vi "I2C_IRQNotifyHost.vi"(8 "error out in":errorcluster, 10 "IRQ Number":u8) -> (0 "error out":errorcluster, 2 "i2c_State":T1)   [LabVIEW 2019]
doc: "Notifies the Host via IRQ that the I2C task has been completed, not that it was successful but that the task has completed executing.\n\n<b>Inputs:</b>\n---------------------\n<b>IRQ Number</b> the IRQ number used for notification.\n0 Write\n1 Read\n3 Write w/Read\n\n<b>Outputs:</b>\n---------------------\n<b>i2c_State</b> hard coded to 'Monitor'\n\nSee block diagram for more details on the implementation details.\n\nAuthor:\nPeter Fuller\nSenior Engineer\nPLF Consulting, LLC\n\nemail: peter@plfconsulting.com\nphone: 617.699.2201"
uses:
  Controls/i2c_state.ctl
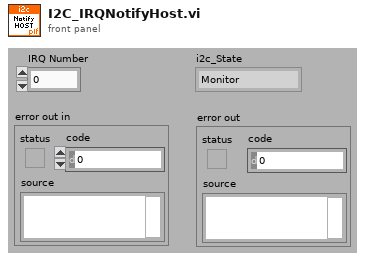
[diagram p1: front panel]
types:
  T1 = typedef "i2c_state.ctl" = enum16{"Monitor", "W_To_Device", "R_From_Device", "W/R_From_Device", "TerminateCore"}
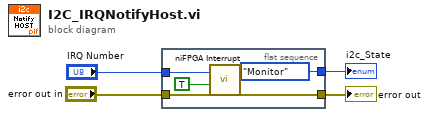
[diagram p0: block diagram]
diagram:
  n1 = flat-sequence {
    tunnel: [i2c_state."Monitor" ("i2c_State")] -> w1
    tunnel: "error out in" -> [w6]
    tunnel: [w6] -> w3
    tunnel: "IRQ Number" -> [w5]
    frame #0 {
      n2 = call <vilib>:"niFPGA Interrupt.vi"("Wait Until Cleared (F)"=TRUE ("Wait Until Cleared"), "IRQ Number (0)"=w5) -> ()  [unwired: 1 in]
    }
  }
  "error out" <- w3
  "i2c_State" <- w1
